vi "Set Pump State.vi"(8 "error in (no error)":errorcluster, 10 "Pump State":bool, 11 "Simulated Evaporative Cooler in":refnum<class "Simulated Evaporative Cooler.lvclass">) -> (0 "error out":errorcluster)   [LabVIEW 2018, in "Simulated Evaporative Cooler.lvclass"]
uses:
  Simulated Evaporative Cooler.lvclass
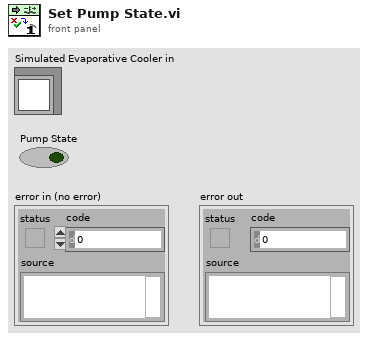
[diagram p1: front panel]
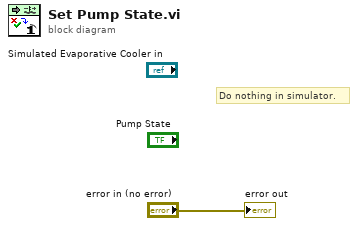
[diagram p0: block diagram]
diagram:
  # "Do nothing in simulator."
  "error out" <- "error in (no error)"
